vi "MB Read_Cached.vi"(8 "error in (no error)":errorcluster, 9 "Quantity(1)":u16=1, 10 "Modbus Reference":u32, 11 "MB PLC in":refnum<class "MB PLC Client.lvclass">) -> (0 "error out":errorcluster, 3 "MB PLC out":refnum<class "MB PLC Client.lvclass">)   [LabVIEW 2018, in "MB PLC Client.lvlib" / "MB PLC Client.lvclass"]
uses:
  MB PLC Client.lvclass
  <vilib>/Plasmionique/MB Master/MB Master.lvlib
  <vilib>/ErrorRing/Error Ring.xnode
  <vilib>/Utility/error.llb/Error Cluster From Error Code.vi
  Data/MB Data Block.lvclass
  MB PLC Client.lvlib
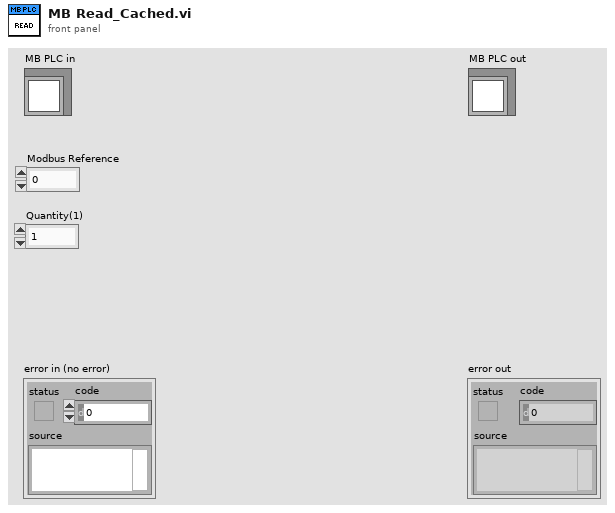
[diagram p1: front panel]
types:
  T1 = typedef "MB PLC Client.lvlib/Reference Types_Enum.ctl" = enum16{"Coil", "Discrete Input", "Input Register", "Holding Register", "Invalid"}
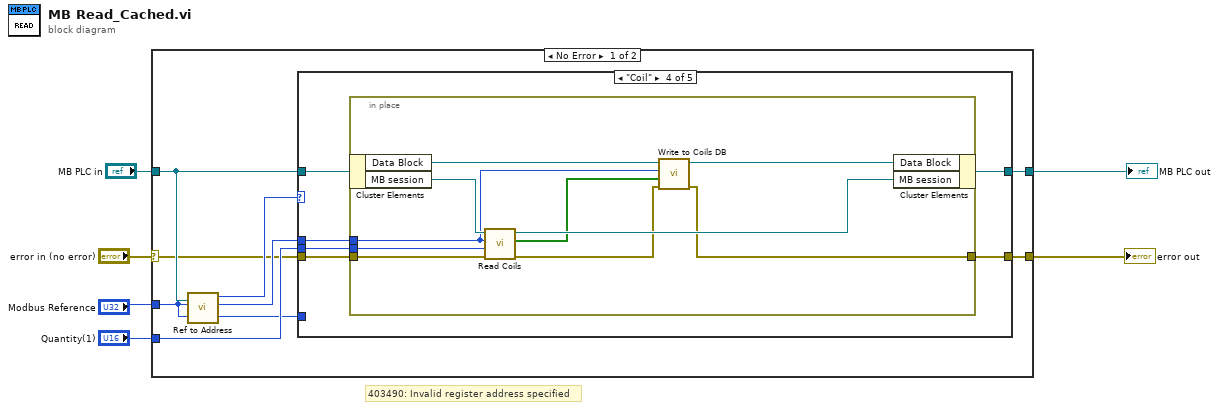
[diagram p0: block diagram]
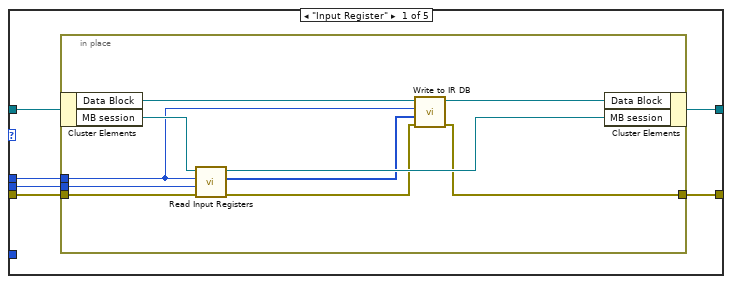
[diagram p2: hidden frame]
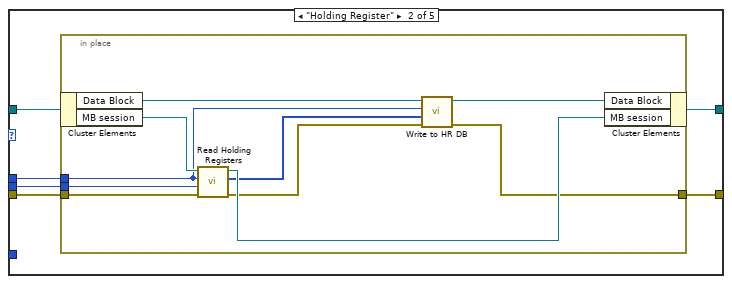
[diagram p3: hidden frame]
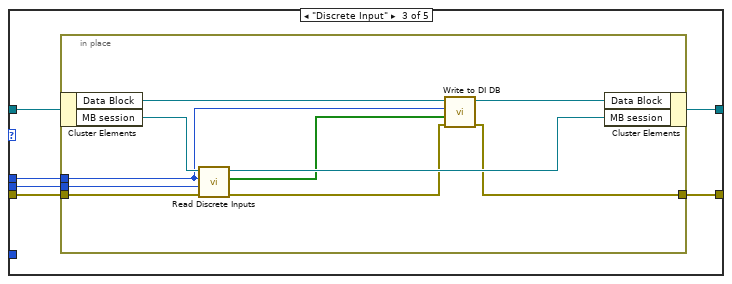
[diagram p4: hidden frame]
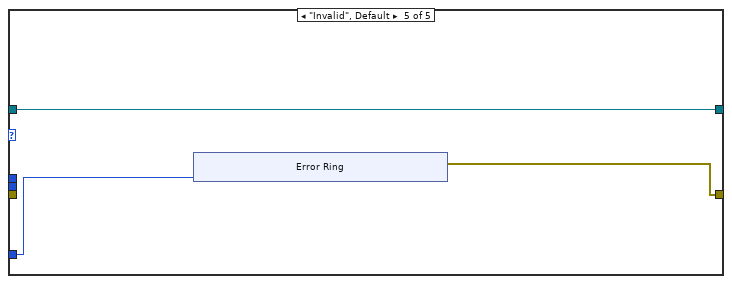
[diagram p5: hidden frame]
diagram:
  # "403490: Invalid register address specified"
  n1 = case shown="No Error" "error in (no error)" {
    selector: "error in (no error)" -> [w8 w89]
    tunnel: [w12 w89] -> w6
    tunnel: "Quantity(1)" -> [w11 _]
    tunnel: "Modbus Reference" -> [w7 _]
    tunnel: "MB PLC in" -> [w10 w90]
    tunnel: [w9 w90] -> w2
    frame No Error {
      n2 = call "Ref to Address.vi"(7:w10, "Reference"=w7) -> ("Address"=w14:u16, "Reference Type"=w13:T1)  [unwired: 8 in]
      n3 = case shown="\"Coil\"" w13 {
        tunnel: w14 -> [w17 w33 w49 w65 _]
        tunnel: w11 -> [w18 w34 w50 w66 _]
        tunnel: w8 -> [w19 w35 w51 w67 _]
        tunnel: [w20 w36 w52 w68 w79] -> w12
        tunnel: w10 -> [w16 w32 w48 w64 w81]
        tunnel: [w15 w31 w47 w63 w81] -> w9
        tunnel: w7 -> [_ _ _ _ w80]
        frame "Input Register" {
          # "Input Reg"
          n4 = in-place {
            in-place-border: [w23] -> w20
            in-place-border: w19 -> [w30]
            in-place-border: w18 -> [w27]
            in-place-border: w17 -> [w22]
            n5 = in-place-cluster #1(w16) -> ("Data Block"=w26:refnum<class "MB Data Block.lvclass">, "MB session"=w29:refnum<class "MB_Master.lvclass">)
            n6 = call <vilib>:"Read Input Registers.vi"("error in (no error)"=w30, "quantity"=w27, "starting address"=w22, "MB session in"=w29) -> ("error out"=w24:errorcluster, "Registers"=w21:u16[], "MB session out"=w28:refnum<class "MB_Master.lvclass">)  [unwired: 5 in]
            n7 = call-dynamic "Write to IR DB.vi"("error in (no error)"=w24, "Values"=w21, "Modbus Address"=w22, "MB Cache in"=w26) -> ("error out"=w23:errorcluster, "MB Cache out"=w25:refnum<class "MB Data Block.lvclass">)  [unwired: 6 in]
            n8 = in-place-cluster #1("Data Block"=w25, "MB session"=w28) -> (w15:refnum<class "MB PLC Client.lvclass">)
          }
        }
        frame "Holding Register" {
          # "Input Reg"
          n9 = in-place {
            in-place-border: [w37] -> w36
            in-place-border: w35 -> [w46]
            in-place-border: w34 -> [w45]
            in-place-border: w33 -> [w39]
            n10 = in-place-cluster #2(w32) -> ("Data Block"=w42:refnum<class "MB Data Block.lvclass">, "MB session"=w44:refnum<class "MB_Master.lvclass">)
            n11 = call <vilib>:"Read Holding Registers.vi"("error in (no error)"=w46, "quantity"=w45, "starting address"=w39, "MB session in"=w44) -> ("error out"=w38:errorcluster, "Registers"=w40:u16[], "MB session out"=w43:refnum<class "MB_Master.lvclass">)  [unwired: 5 in]
            n12 = call-dynamic "Write to HR DB.vi"("error in (no error)"=w38, "Values"=w40, "Modbus Address"=w39, "MB Cache in"=w42) -> ("error out"=w37:errorcluster, "MB Cache out"=w41:refnum<class "MB Data Block.lvclass">)  [unwired: 6 in]
            n13 = in-place-cluster #2("Data Block"=w41, "MB session"=w43) -> (w31:refnum<class "MB PLC Client.lvclass">)
          }
        }
        frame "Discrete Input" {
          # "Input Reg"
          n14 = in-place {
            in-place-border: [w55] -> w52
            in-place-border: w51 -> [w61]
            in-place-border: w50 -> [w60]
            in-place-border: w49 -> [w53]
            n15 = in-place-cluster #3(w48) -> ("Data Block"=w58:refnum<class "MB Data Block.lvclass">, "MB session"=w62:refnum<class "MB_Master.lvclass">)
            n16 = call <vilib>:"Read Discrete Inputs.vi"("error in (no error)"=w61, "quantity"=w60, "starting address"=w53, "MB session in"=w62) -> ("error out"=w56:errorcluster, "Inputs"=w54:bool[], "MB session out"=w59:refnum<class "MB_Master.lvclass">)  [unwired: 5 in]
            n17 = call-dynamic "Write to DI DB.vi"("error in (no error)"=w56, "Values"=w54, "Modbus Address"=w53, "MB Cache in"=w58) -> ("error out"=w55:errorcluster, "MB Cache out"=w57:refnum<class "MB Data Block.lvclass">)  [unwired: 6 in]
            n18 = in-place-cluster #3("Data Block"=w57, "MB session"=w59) -> (w47:refnum<class "MB PLC Client.lvclass">)
          }
        }
        frame "Coil" {
          # "Input Reg"
          n19 = in-place {
            in-place-border: [w72] -> w68
            in-place-border: w67 -> [w78]
            in-place-border: w66 -> [w77]
            in-place-border: w65 -> [w69]
            n20 = in-place-cluster #4(w64) -> ("Data Block"=w74:refnum<class "MB Data Block.lvclass">, "MB session"=w76:refnum<class "MB_Master.lvclass">)
            n21 = call <vilib>:"Read Coils.vi"("error in (no error)"=w78, "quantity"=w77, "starting address"=w69, "MB session in"=w76) -> ("error out"=w73:errorcluster, "Coils"=w70:bool[], "MB session out"=w75:refnum<class "MB_Master.lvclass">)  [unwired: 5 in]
            n22 = call-dynamic "Write to Coils DB.vi"("error in (no error)"=w73, "Values"=w70, "Modbus Address"=w69, "MB Cache in"=w74) -> ("error out"=w72:errorcluster, "MB Cache out"=w71:refnum<class "MB Data Block.lvclass">)  [unwired: 6 in]
            n23 = in-place-cluster #4("Data Block"=w71, "MB session"=w75) -> (w63:refnum<class "MB PLC Client.lvclass">)
          }
        }
        frame "Invalid", Default {
          # "Invalid"
          n24 = xnode "Error Ring"("parameter 0"=w80) -> ("error out"=w79:errorcluster)
        }
      }
    }
    frame Error {
    }
  }
  "error out" <- w6
  "MB PLC out" <- w2
